vi "VIQA Audit VI.vi"(6 "Pwrd Skip All? (F)":bool, 8 "error in (no error)":errorcluster, 9 "Ignore":T2, 10 "Item ID":string, 11 "VI Refnum":refnum<vi>) -> (0 "error out":errorcluster, 1 "Valid?":bool, 2 "Item":T1, 3 "dup VI Refnum":refnum<vi>, 4 "Pwrd Skip All?":bool)   [LabVIEW 2018, in "VI Quality.lvlib"]
uses:
  VI Quality.lvlib
  Controls/VIQA Audit.ctl
  Controls/VIQA Audit Ignore.ctl
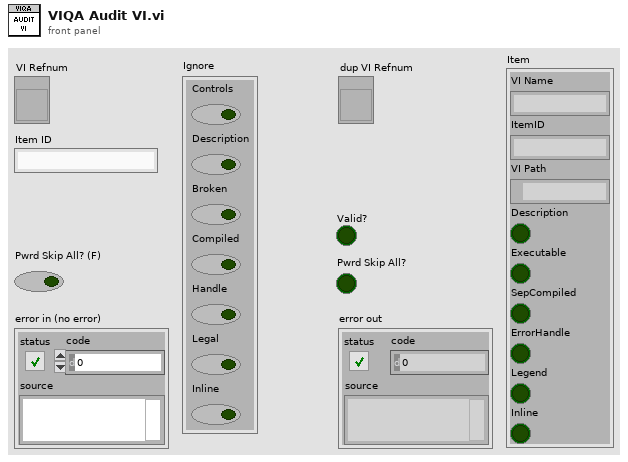
[diagram p1: front panel]
types:
  T1 = typedef "VI Quality.lvlib/VIQA Audit.ctl" = cluster{"VI Name":string, "ItemID":string, "VI Path":path, "Description":bool, "Executable":bool, "SepCompiled":bool, "ErrorHandle":bool, "Legend":bool, "Inline":bool}
  T2 = typedef "VI Quality.lvlib/VIQA Audit Ignore.ctl" = cluster{"Controls":bool, "Description":bool, "Broken":bool, "Compiled":bool, "Handle":bool, "Legal":bool, "Inline":bool}
  T3 = enum32{"Bad", "Idle", "Run top level", "Running"}
  T4 = enum32{"invalid VI type", "Standard VI", "Control VI", "Global VI", "Polymorphic VI", "Configuration VI", "SubSystem", "Facade VI", "Method VI", "Statechart Diagram VI"}
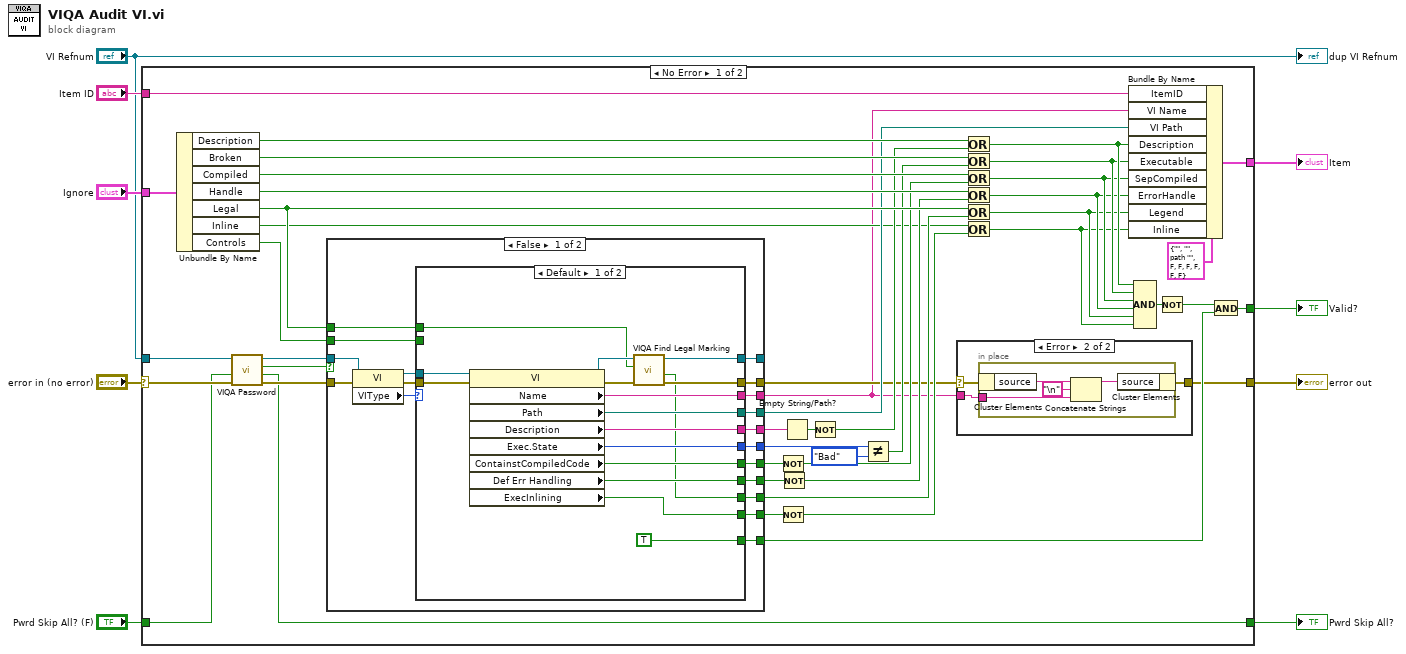
[diagram p0: block diagram]
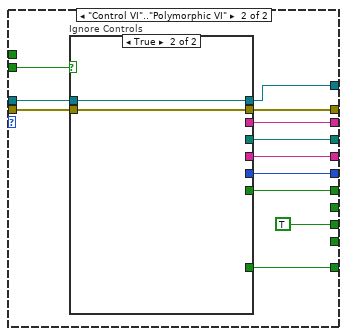
[diagram p3: hidden frame]
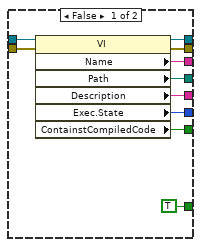
[diagram p4: hidden frame]
diagram:
  n1 = case shown="No Error" "error in (no error)" {
    selector: "error in (no error)" -> [w47 w124]
    tunnel: "Ignore" -> [w54 _]
    tunnel: "VI Refnum" -> [w48 _]
    tunnel: "Item ID" -> [w46 _]
    tunnel: "Pwrd Skip All? (F)" -> [w21 w123]
    tunnel: [w20 _] -> w5
    tunnel: [w19 _] -> w4
    tunnel: [w11 w124] -> w3
    tunnel: [w14 w123] -> w2
    frame No Error {
      n2 = Unbundle By Name(w54) -> ("Description"=w53:bool, "Broken"=w52:bool, "Compiled"=w51:bool, "Handle"=w50:bool, "Legal"=w49:bool, "Inline"=w17:bool, "Controls"=w13:bool)
      n3 = call "VIQA Password.vi"("error in (no error)"=w47, "Skip All? (F)"=w21, "VI Refnum"=w48) -> ("error out"=w24:errorcluster, "Skip All?"=w14:bool, "Locked"=w22:bool, "dup VI Refnum"=w23:refnum<vi>)  [unwired: 5 in]
      n4 = case shown="False" w22 {
        tunnel: [w80 _] -> w45
        tunnel: [w79 _] -> w42
        tunnel: [w78 _] -> w10
        tunnel: [w77 _] -> w40
        tunnel: [w76 _] -> w39
        tunnel: [w75 _] -> w38
        tunnel: w13 -> [w71 _]
        tunnel: [w70 _] -> w27
        tunnel: [w69 w122] -> w12
        tunnel: [w68 _] -> w26
        tunnel: [w67 w121] -> _
        tunnel: w49 -> [w66 _]
        tunnel: w24 -> [w65 w122]
        tunnel: w23 -> [w64 w121]
        tunnel: [w63 _] -> w18
        frame False {
          n5 = property class="VI"(reference=w64, error in=w65) -> (reference out=w72:refnum<vi>, error out=w74:errorcluster, "VIType"=w73:T4)
          n6 = case shown="Default" w73 {
            tunnel: [w85 w108] -> w69
            tunnel: [w84 w107] -> w67
            tunnel: [w96 w106] -> w80
            tunnel: [w95 w105] -> w79
            tunnel: [w94 w104] -> w78
            tunnel: [w93 w103] -> w77
            tunnel: [w92 w102] -> w76
            tunnel: [w91 _] -> w75
            tunnel: w74 -> [w90 w101]
            tunnel: w72 -> [w89 w100]
            tunnel: [TRUE w97] -> w70
            tunnel: w71 -> [_ w99]
            tunnel: [w83 TRUE ("Found?")] -> w68
            tunnel: w66 -> [w82 _]
            tunnel: [w81 _] -> w63
            frame Default {
              n7 = property class="VI"(reference=w89, error in=w90) -> (reference out=w86:refnum<vi>, error out=w87:errorcluster, "Name"=w94:string, "Path"=w93:path, "Description"=w96:string, "Exec.State"=w95:T3, "ContainstCompiledCode"=w92:bool, "Def Err Handling"=w91:bool, "ExecInlining"=w81:bool)
              n8 = call "VIQA Find Legal Marking.vi"("error in (no error)"=w87, "Ignore? (F)"=w82, "VI Refnum"=w86) -> ("error out"=w85:errorcluster, "Found?"=w83:bool, "dup VI Refnum"=w84:refnum<vi>)  [unwired: 3 in, 3 out]
            }
            frame "Control VI".."Polymorphic VI" {
              n9 = case "Ignore Controls" shown="True" w99 {
                tunnel: [w118 w120] -> w108
                tunnel: [w117 w119] -> w107
                tunnel: [w116 _] -> w106
                tunnel: [w115 _] -> w105
                tunnel: [w114 _] -> w104
                tunnel: [w113 _] -> w103
                tunnel: [w112 _] -> w102
                tunnel: w101 -> [w111 w120]
                tunnel: w100 -> [w110 w119]
                tunnel: [TRUE _] -> w97
                frame False {
                  n10 = property class="VI"(reference=w110, error in=w111) -> (reference out=w117:refnum<vi>, error out=w118:errorcluster, "Name"=w114:string, "Path"=w113:path, "Description"=w116:string, "Exec.State"=w115:T3, "ContainstCompiledCode"=w112:bool)
                }
                frame True {
                }
              }
            }
          }
        }
        frame True {
        }
      }
      n11 = Not(x=w39) -> (.not. x?=w35:bool)
      n12 = Not(x=w18) -> (.not. x?=w16:bool)
      n13 = Not(x=w38) -> (.not. x?=w34:bool)
      n14 = Empty String/Path?(string/path=w45) -> (empty?=w44:bool)
      n15 = Not(x=w44) -> (.not. x?=w37:bool)
      n16 = Not Equal?(x=w42, y=T3."Bad") -> (x != y?=w36:bool)
      n17 = case shown="Error" w12 {
        selector: w12 -> [w55 w58]
        tunnel: [w55 w57] -> w11
        tunnel: w10 -> [_ w56]
        frame No Error {
        }
        frame Error {
          n18 = in-place {
            in-place-border: w56 -> [w60]
            n19 = in-place-cluster #1(w58) -> ("source"=w62:string)
            n20 = Concatenate Strings(w62, "\n" ("Line Feed Constant"), w60) -> (w61:string)
            n21 = in-place-cluster #1("source"=w61) -> (w57:errorcluster)
          }
        }
      }
      n22 = Or(x=w53, y=w37) -> (x .or. y?=w32:bool)
      n23 = Or(x=w52, y=w36) -> (x .or. y?=w31:bool)
      n24 = Or(x=w51, y=w35) -> (x .or. y?=w30:bool)
      n25 = Or(x=w50, y=w34) -> (x .or. y?=w29:bool)
      n26 = Or(x=w49, y=w26) -> (x .or. y?=w25:bool)
      n27 = Or(x=w17, y=w16) -> (x .or. y?=w15:bool)
      n28 = Bundle By Name(cluster=T1 {"VI Name"="", "ItemID"="", "VI Path"=path "", "Description"=FALSE, "Executable"=FALSE, "SepCompiled"=FALSE, "ErrorHandle"=FALSE, "Legend"=FALSE, "Inline"=FALSE} ("Audit"), "ItemID"=w46, "VI Name"=w10, "VI Path"=w40, "Description"=w32, "Executable"=w31, "SepCompiled"=w30, "ErrorHandle"=w29, "Legend"=w25, "Inline"=w15) -> (w19:T1)
      n29 = Compound Arithmetic op=AND(w32, w31, w30, w29, w25, w15) -> (w33:bool)
      n30 = Not(x=w33) -> (.not. x?=w28:bool)
      n31 = And(x=w28, y=w27) -> (x .and. y?=w20:bool)
    }
    frame Error {
    }
  }
  "error out" <- w3
  "Pwrd Skip All?" <- w2
  "Valid?" <- w5
  "Item" <- w4
  "dup VI Refnum" <- "VI Refnum"
